vi "Destroy Object Buffer.vi"(8 "error in":errorcluster, 9 "Return Elements (T)":bool=TRUE, 11 "Buffer":refnum<data-value>) -> (0 "error out":errorcluster, 2 "elements":refnum<class>[](array[class]))   [LabVIEW 2013, in "CircularBuffer.lvlib" / "ObjectBuffer.lvclass"]
doc: "This VI releases resources that have been created for the ring buffer."
uses:
  ObjectBuffer.lvclass
  VariantBuffer/VariantBuffer.lvclass
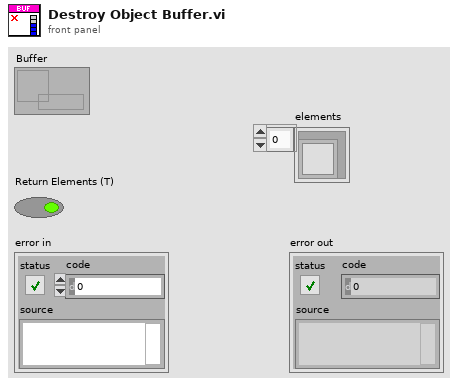
[diagram p1: front panel]
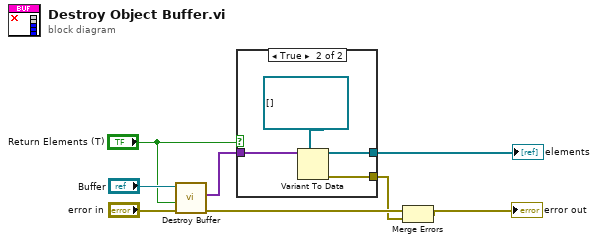
[diagram p0: block diagram]
diagram:
  n1 = call "Destroy Buffer.vi"("error in"="error in", "Return Elements (T)"="Return Elements (T)", "Buffer"="Buffer") -> ("error out"=w7:errorcluster, "elements"=w8:variant[])  [unwired: 7 in]
  n2 = case shown="True" "Return Elements (T)" {
    tunnel: [_ w11] -> w2
    tunnel: w8 -> [_ w12]
    tunnel: [_ w10] -> w6
    frame False {
    }
    frame True {
      n3 = Variant To Data(type=refnum<class>[] [] ("elements"), Variant=w12) -> (data=w11:refnum<class>[], error out=w10:errorcluster)  [unwired: 1 in]
    }
  }
  "elements" <- w2
  n4 = Merge Errors(w7, w6) -> (→"error out":errorcluster)
